vi "SearchPage.vi"() -> ()   [LabVIEW 2016]
uses:
  <resource>/dialog/NewProjectWizard/MetaDataObj/MetaDataObj.lvclass
  <resource>/dialog/NewProjectWizard/Operation to Log.ctl
  <resource>/dialog/NewProjectWizard/MetaDataObj/Accessors/Read Documentation Path.vi
  <vilib>/Platform/browser.llb/Open URL in Default Browser (path).vi
  <resource>/dialog/NewProjectWizard/MetaDataObj/Accessors/Read Custom VI Mode.vi
  <resource>/dialog/NewProjectWizard/Loading Project Info/NI_NPW_Loading Project Info.lvlib
  <resource>/dialog/NewProjectWizard/Filters/NI_NPW_Filters.lvlib
panel:
  in  "Next":string="下一步" caption="下一步"
  in  "Finish":string="完成" caption="完成"
  in  "Filters":string(tree)="All" caption="过滤"
  in  "Main Next":refnum<vi> caption="主界面下一步"
  in  "Additional Search":string caption="附加搜索"
  in  "Project List":picture caption="项目列表"
  out "Go To Next Page":bool caption="转至下一页"
  in  "Tab Backward To":refnum<vi> caption="按Tab后退至"
  in  "Tab Forward To":refnum<vi> caption="按Tab前进至"
  in  "Default Searchbox Text":string="关键词" caption="默认搜索框文本"
  out "Current Starter Application":refnum<class "MetaDataObj.lvclass"> caption="当前启动应用程序"
  in  "Scrollbar":i32(c297) caption="滚动条"
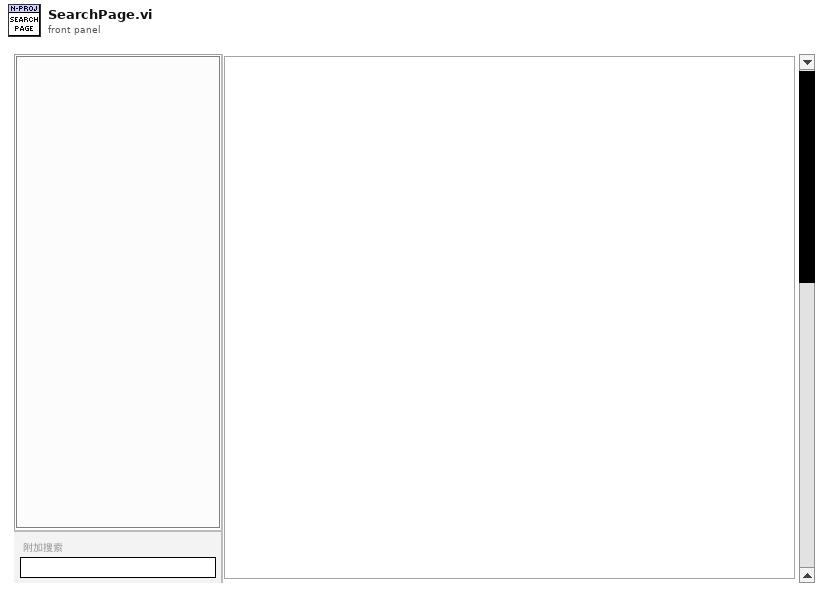
[diagram p1: front panel]
types:
  T1 = typedef "Operation to Log.ctl" = enum16{"Create", "Cancel", "MoreInfoLink"}
  T2 = enum8{"Enabled", "Disabled", "Disabled and Grayed Out"}
  T3 = typedef "imagedata.ctl" = cluster{"image type":i32, "image depth":i32, "image":u8[], "mask":u8[], "colors":u32[], "Rectangle":cluster{"left":i16, "top":i16, "right":i16, "bottom":i16}}
  T4 = typedef "LVBoundsTypeDef.ctl" = cluster{"Width":u32, "Height":u32}
  T5 = typedef "eventvkey.ctl" = enum16{"ASCII", "Enter", "Return", "Shift", "Ctrl", "Alt", "Cmd", "Opt", "Caps", "NumLock", "Clear", "Break", "Up", "Down", "Left", "Right", "Insert", "Delete", "Home", "End", "PageUp", "PageDown", "Escape", "Help", "Pause", "ScrollLock", "F1", "F2", "F3", "F4", "F5", "F6", "F7", "F8", "F9", "F10", "F11", "F12", "F13", "F14", "F15", "F16", "F17", "F18", "F19", "F20", "F21", "F22", "F23", "F24", "Play", "VolumeUp", "VolumeDown", "Mute", "Two Byte Char"}
  T6 = typedef "CustomVIModes.ctl" = enum16{"None", "AfterPage1", "AfterPage2WithUI", "AfterPage2NoUI"}
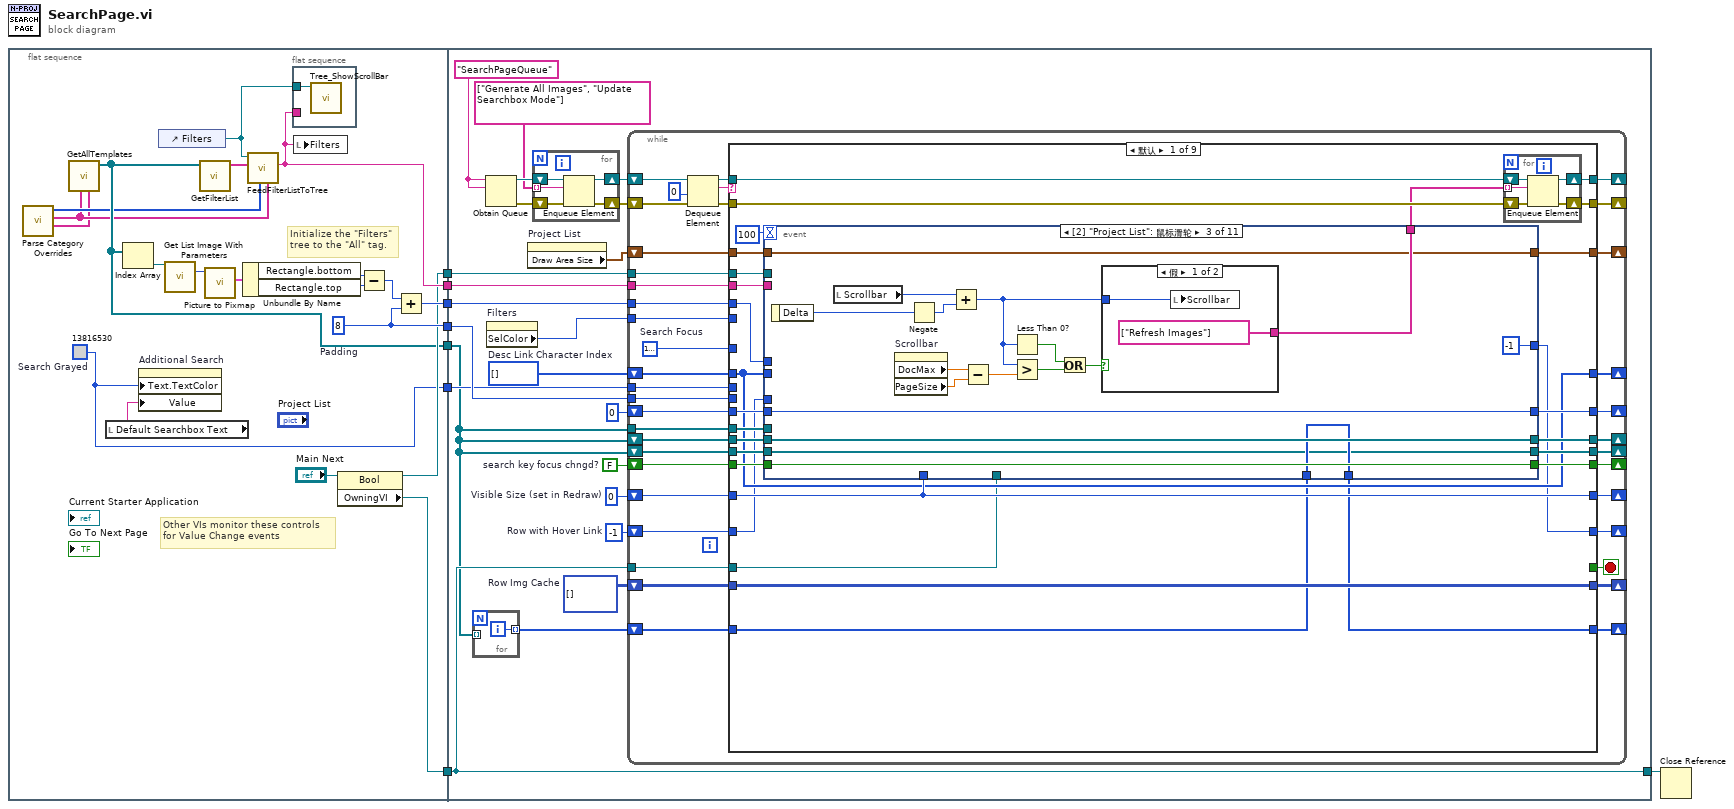
[diagram p0: block diagram]
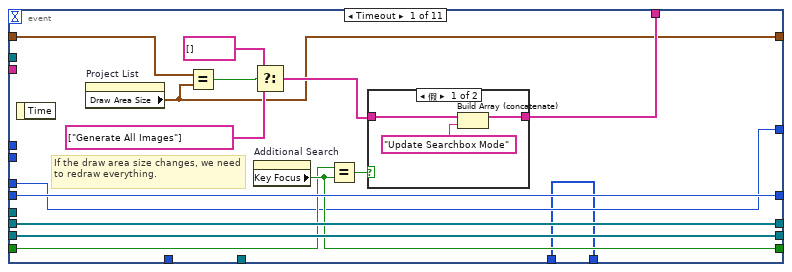
[diagram p2: hidden frame]
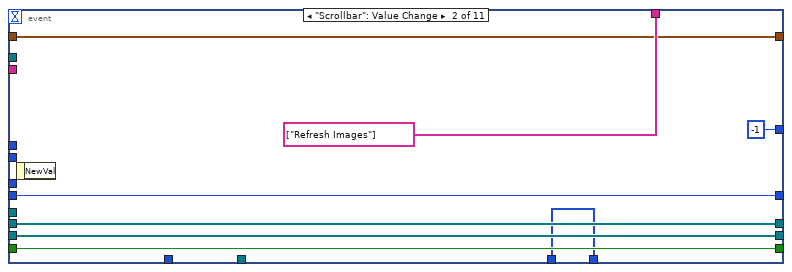
[diagram p4: hidden frame]
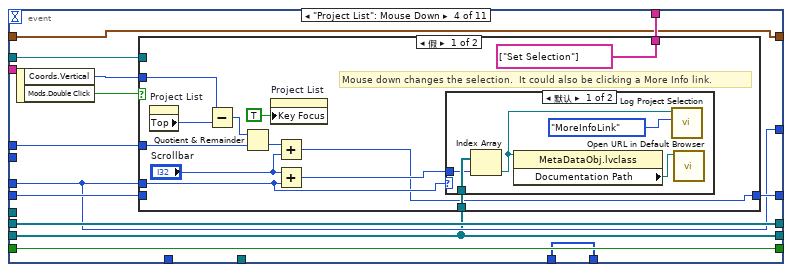
[diagram p6: hidden frame]
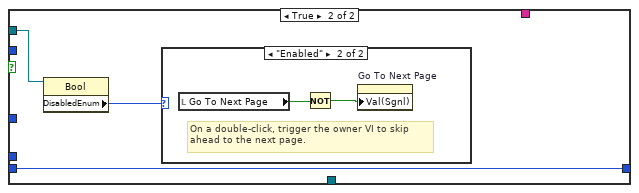
[diagram p8: hidden frame]
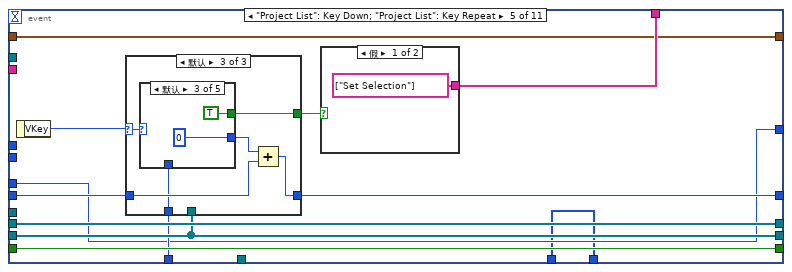
[diagram p10: hidden frame]
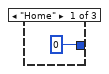
[diagram p12: hidden frame]
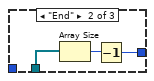
[diagram p13: hidden frame]
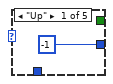
[diagram p14: hidden frame]
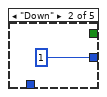
[diagram p15: hidden frame]
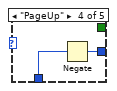
[diagram p16: hidden frame]
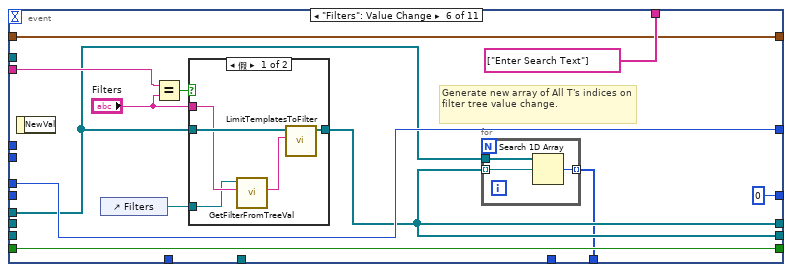
[diagram p18: hidden frame]
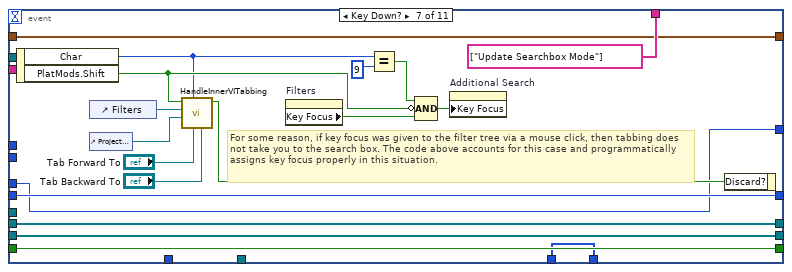
[diagram p20: hidden frame]
diagram:
  n1 = flat-sequence {
    tunnel: [w13] -> w8
    tunnel: [w20] -> w7
    tunnel: [w21] -> w6
    tunnel: [w18] -> w5
    tunnel: [w16] -> w4
    tunnel: [w15] -> w3
    tunnel: [w12] -> w1
    tunnel: w8 -> [w31]
    tunnel: w7 -> [w50]
    tunnel: w6 -> [w49]
    tunnel: w5 -> [w45]
    tunnel: w4 -> [w40]
    tunnel: w3 -> [w39]
    tunnel: [w39] -> w2
    tunnel: w1 -> [w38]
    frame #0 {
      w12 = u32 13816530  # Search Grayed
      w21 = i8 8  # Padding
      # "Other VIs monitor these controls\nfor Value Change events"
      # "Initialize the \"Filters\"\ntree to the \"All\" tag."
      n2 = call <resource>:"Parse Category Overrides.vi"() -> ("Non Localized Names"=w9:string[], "Names"=w10:string[], "Priorities"=w11:i32[])  [unwired: 9 in]
      n3 = call <resource>:"GetAllTemplates.vi"("Category Nonlocalized Names"=w9, "Category Names"=w10) -> ("Templates Out"=w13:refnum<class "MetaDataObj.lvclass">[])  [unwired: 9 in]
      n4 = local read "Default Searchbox Text"() -> (w14:string)
      n5 = Index Array(array=w13) -> (element=w28:refnum<class "MetaDataObj.lvclass">)  [unwired: 1 in]
      n6 = property on="Additional Search" class="Str"("Text.TextColor"=w12, "Value"=w14) -> ()  [unwired: 2 in, 2 out]
      n7 = control-ref of="Filters"() -> (w19:refnum<vi>)
      n8 = call <resource>:"Get List Image With Parameters.vi"("Template in"=w28) -> ("Image"=w27:picture)  [unwired: 10 in, 4 out]
      n9 = call <resource>:"GetFilterList.vi"("Templates"=w13) -> ("Filters"=w23:string[])  [unwired: 10 in]
      n10 = call <vilib>:"Picture to Pixmap.vi"("picture"=w27) -> ("image data"=w26:T3)  [unwired: 9 in, 1 out]
      n11 = Unbundle By Name(w26) -> ("Rectangle.bottom"=w25:i16, "Rectangle.top"=w24:i16)
      n12 = call <resource>:"FeedFilterListToTree.vi"("Category Names"=w10, "Category Priorities"=w11, "Filters"=w23, "Tree Ref In"=w19) -> ("\"All\" Tag"=w20:string)  [unwired: 6 in, 1 out]
      n13 = flat-sequence {
        tunnel: w20 -> [_]
        tunnel: w19 -> [w29]
        frame #0 {
          n14 = call <vilib>:"Tree_ShowScrollBar.vi"("Tree"=w29) -> ()  [unwired: 10 in, 1 out]
        }
      }
      n15 = local write "Filters"(w20) -> ()
      n16 = property class="Bool"(reference="Main Next") -> (reference out=w16:refnum<vi>, "OwningVI"=w15:refnum<vi>)  [unwired: 1 in, 1 out]
      n17 = Subtract(x=w25, y=w24) -> (x-y=w22:i16)
      n18 = Add(x=w22, y=w21) -> (x+y=w18:i16)
    }
    frame #1 {
      w37 = picture[][] []  # Row Img Cache
      w42 = -1  # Row with Hover Link
      w43 = i32[] []  # Desc Link Character Index
      w44 = i8 0  # Visible Size (set in Redraw)
      w46 = FALSE  # search key focus chngd?
      w34 = "SearchPageQueue" ("name (unnamed)")
      n19 = for {
        tunnel: [w52] -> w32 mode=indexing
        tunnel: w31 -> [_] mode=indexing
        i -> [w52]
      }
      n20 = Obtain Queue(name (unnamed)=w34, element data type=w34) -> (queue out=w35:refnum<queue>, error out=w36:errorcluster)  [unwired: 3 in, 1 out]
      n21 = property on="Filters" class="Tree (严格)"() -> ("SelColor"=w41:u32)  [unwired: 2 in, 2 out]
      n22 = property on="Project List" class="Pict"() -> ("Draw Area Size"=w30:T4)  [unwired: 2 in, 2 out]
      n23 = for {
        shift-right: [w57] -> w48
        shift-left: w35 -> [w54]
        shift-right: [w56] -> w47
        shift-left: w36 -> [w55]
        tunnel: string[] ["Generate All Images", "Update Searchbox Mode"] -> [w53] mode=indexing
        n24 = Enqueue Element(queue=w54, element=w53, error in (no error)=w55) -> (queue out=w57:refnum<queue>, error out=w56:errorcluster)  [unwired: 1 in, 1 out]
      }
      n25 = while {
        shift-right: [w90] -> _
        shift-left: w47 -> [w94]
        shift-right: [w78] -> _
        shift-left: w48 -> [w95]
        tunnel: w31 -> [w87]
        shift-right: [w83] -> _
        shift-left: w31 -> [w86]
        shift-right: [w84] -> _
        shift-left: w31 -> [w85]
        shift-right: [w81] -> _
        shift-left: 0 ("Selection") -> [w82]
        tunnel: w50 -> [w80]
        tunnel: w49 -> [w79]
        shift-right: [w75] -> _
        shift-left: w46 -> [w76]
        tunnel: w45 -> [w74]
        shift-right: [w72] -> _
        shift-left: w44 -> [w73]
        shift-right: [w71] -> _
        shift-left: w43 -> [w70]
        shift-right: [w68] -> _
        shift-left: w42 -> [w69]
        tunnel: w41 -> [w67]
        tunnel: w40 -> [w66]
        tunnel: w39 -> [w65]
        tunnel: w38 -> [w64]
        shift-right: [w62] -> _
        shift-left: w37 -> [w63]
        shift-right: [w60] -> _
        shift-left: w32 -> [w61]
        shift-right: [w58] -> _
        shift-left: w30 -> [w59]
        stop <- w88 stop-if-true
        w77 = u32 16777222  # Search Focus
        n26 = Dequeue Element(queue=w95, timeout in ms (-1)=0, error in (no error)=w94) -> (queue out=w93:refnum<queue>, element=w91:string, error out=w92:errorcluster)  [unwired: 1 out]
        n27 = case shown="默认" w91 {
          tunnel: w93 -> [w114 w354 w389 w430 w464 w496 w516 w546 w577]
          tunnel: w92 -> [w113 w351 w400 w429 w462 w497 w515 w545 w576]
          tunnel: [w112 w352 w390 w429 w461 w487 w515 w545 w576] -> w90
          tunnel: [_ _ _ _ _ _ _ _ TRUE] -> w88
          tunnel: w87 -> [w118 _ w385 _ w443 _ _ _ _]
          tunnel: w86 -> [w122 w349 w396 w428 w454 w492 w514 w552 w575]
          tunnel: w85 -> [w120 w348 w395 w427 w455 w491 w513 w551 w574]
          tunnel: [w119 w348 w395 w427 w442 w491 w513 w551 w574] -> w84
          tunnel: [w121 w349 w396 w428 w454 w492 w514 w552 w575] -> w83
          tunnel: w82 -> [w117 w347 w394 w426 _ w490 w512 w550 w573]
          tunnel: [w116 w347 w394 w426 0 ("lower limit") w489 w512 w550 w573] -> w81
          tunnel: w80 -> [w115 _ _ _ _ _ _ _ _]
          tunnel: w79 -> [_ w346 _ _ _ _ _ _ _]
          tunnel: [w110 w353 w388 w430 w463 w488 w516 w546 w577] -> w78
          tunnel: w77 -> [_ _ _ _ w457 _ _ w544 _]
          tunnel: w76 -> [w109 w345 w393 w425 w453 w486 w511 w543 w572]
          tunnel: [w108 w345 w393 w425 w453 w486 w511 w543 w572] -> w75
          tunnel: w74 -> [w107 w344 _ w424 _ _ _ _ _]
          tunnel: w73 -> [w106 _ w383 w423 w452 w485 w510 w542 w571]
          tunnel: [w106 w343 w383 w423 w452 w485 w510 w542 w571] -> w72
          tunnel: [w105 w331 w382 w422 w451 w484 w509 w541 w570] -> w71
          tunnel: w70 -> [w105 w331 _ w422 w451 w484 w509 w541 w570]
          tunnel: w69 -> [w104 w342 w392 w421 w450 w483 w508 w540 w569]
          tunnel: [w103 w342 w392 w421 w450 w483 w508 w540 w569] -> w68
          tunnel: w66 -> [w101 _ _ _ w448 w480 _ _ _]
          tunnel: w67 -> [_ _ w391 _ _ _ _ _ _]
          tunnel: w65 -> [w102 _ _ _ _ _ _ _ _]
          tunnel: w64 -> [_ _ _ _ _ _ _ w539 _]
          tunnel: w63 -> [w100 w333 _ w419 w444 w478 w507 w538 w568]
          tunnel: [w100 w333 w384 w419 w444 w478 w507 w538 w568] -> w62
          tunnel: w61 -> [w99 w332 w386 w418 _ w477 w506 w537 w567]
          tunnel: [w98 w332 w386 w418 w441 w477 w506 w537 w567] -> w60
          tunnel: w59 -> [w97 w325 w381 w417 w440 w476 w505 w536 w566]
          tunnel: [w96 w325 w381 w417 w440 w476 w505 w536 w566] -> w58
          frame Default {
            n28 = event shown="[2] \"Project List\": 鼠标滑轮" {
              selector: _ -> [_ _ _ _ _ _ _ _ _ _ _]
              dyn-events: _ -> [_ _ _ _ _ _ _ _ _ _ _]
              timeout: 100 -> [_ _ _ _ _ _ _ _ _ _ _]
              tunnel: [w137 string[] ["Refresh Images"] w171 w183 w216 string[] ["Enter Search Text"] string[] ["Update Searchbox Mode"] string[] ["Update Searchbox Mode"] w299 w309 string[] ["Update Searchbox Mode"]] -> w111
              tunnel: w122 -> [w143 w155 w173 w186 w220 _ w277 w287 w294 w316 w324]
              tunnel: [w143 w155 w173 w186 w220 w243 w277 w287 w294 w316 w324] -> w121
              tunnel: [w142 w154 w165 w179 w219 w243 w276 w286 w293 w306 w323] -> w119
              tunnel: w120 -> [w142 w154 w165 w179 w219 _ w276 w286 w293 w306 w323]
              tunnel: w118 -> [_ _ _ _ _ w244 _ _ _ _ _]
              tunnel: w117 -> [w141 w153 w172 w184 w217 _ w275 w288 w295 w315 w322]
              tunnel: [w141 w153 w172 w185 w218 0 ("Selection") w275 w288 w295 w315 w322] -> w116
              tunnel: w115 -> [_ _ _ _ _ w249 _ _ _ _ _]
              tunnel: w109 -> [w139 w151 w170 w182 w215 w247 w273 w285 w292 w314 w320]
              tunnel: [w140 w151 w170 w182 w215 w247 w273 w285 w292 w314 w320] -> w108
              tunnel: w107 -> [_ _ _ w181 _ _ _ _ _ w304 _]
              tunnel: w106 -> [_ _ _ _ w214 _ _ _ _ _ _]
              tunnel: w105 -> [_ _ _ _ _ _ _ _ _ w305 _]
              tunnel: w104 -> [w136 _ _ w180 w213 w245 w270 w284 w291 w307 w319]
              tunnel: [w136 -1 ("Row with Hover Link") -1 ("Row with Hover Link") w180 w213 w245 w270 w284 w291 w308 w319] -> w103
              tunnel: w102 -> [_ _ _ _ _ _ _ _ _ w303 _]
              tunnel: w101 -> [_ _ _ w178 _ _ _ _ _ _ _]
              tunnel: w99 -> [w135 w149 w168 w177 w212 _ w269 w283 w290 w302 w318]
              tunnel: [w135 w149 w168 w177 w212 w242 w269 w283 w290 w302 w318] -> w98
              tunnel: w97 -> [w134 w148 w167 w176 w211 w241 w268 w282 w289 w301 w317]
              tunnel: [w129 w148 w167 w176 w211 w241 w268 w282 w289 w301 w317] -> w96
              event Timeout {
                # "If the draw area size changes, we need to redraw everything."
                n29 = event-data() -> ()  [unwired: 1 in, 1 out]
                n30 = property on="Project List" class="Pict"() -> ("Draw Area Size"=w129:T4)  [unwired: 2 in, 2 out]
                n31 = Equal?(x=w134, y=w129) -> (x = y?=w133:bool)
                n32 = property on="Additional Search" class="Str"() -> ("Key Focus"=w140:bool)  [unwired: 2 in, 2 out]
                n33 = Select(t=string[] [], s=w133, f=string[] ["Generate All Images"]) -> (s? t:f=w131:string[])
                n34 = Equal?(x=w139, y=w140) -> (x = y?=w138:bool)
                n35 = case shown="假" w138 {
                  tunnel: w131 -> [w146 w147]
                  tunnel: [w145 w147] -> w137
                  frame False {
                    n36 = Build Array (concatenate)(w146, "Update Searchbox Mode") -> (w145:string[])
                  }
                  frame True {
                  }
                }
              }
              event "Scrollbar": Value Change {
                n37 = event-data() -> ()  [unwired: 1 in, 1 out]
              }
              event "Project List": Mouse Wheel {
                n38 = event-data() -> ("Delta"=w166:i32)  [unwired: 1 in]
                n39 = local read "Scrollbar"() -> (w163:i32)
                n40 = property on="Scrollbar" class="Scroll (严格)"() -> ("DocMax"=w158:dbl, "PageSize"=w157:dbl)  [unwired: 2 in, 2 out]
                n41 = Negate(x=w166) -> (-x=w161:i32)
                n42 = Add(x=w163, y=w161) -> (x+y=w160:i32)
                n43 = Subtract(x=w158, y=w157) -> (x-y=w156:dbl)
                n44 = Less Than 0?(x=w160) -> (x < 0?=w162:bool)
                n45 = Greater?(x=w160, y=w156) -> (0:w164:bool)
                n46 = Or(x=w162, y=w164) -> (x .or. y?=w159:bool)
                n47 = case shown="假" w159 {
                  tunnel: [string[] ["Refresh Images"] _] -> w171
                  tunnel: w160 -> [w174 _]
                  frame False {
                    n48 = local write "Scrollbar"(w174) -> ()
                  }
                  frame True {
                  }
                }
              }
              event "Project List": Mouse Down {
                n49 = event-data() -> ("Coords.Vertical"=w188:i32, "Mods.Double Click"=w187:bool)  [unwired: 1 in]
                n50 = case shown="假" w187 {
                  tunnel: w188 -> [w200 _]
                  tunnel: [w189 w208] -> w185
                  tunnel: w184 -> [_ w208]
                  tunnel: [string[] ["Set Selection"] _] -> w183
                  tunnel: w181 -> [w194 _]
                  tunnel: w180 -> [w190 _]
                  tunnel: w179 -> [w193 _]
                  tunnel: w178 -> [_ w207]
                  frame False {
                    # "Mouse down changes the selection.  It could also be clicking a More Info link."
                    n51 = property on="Project List" class="Pict"() -> ("Top"=w199:i32)  [unwired: 2 in, 2 out]
                    n52 = Subtract(x=w200, y=w199) -> (x-y=w198:i32)
                    n53 = Quotient & Remainder(x=w198, y=w194) -> (floor(x/y)=w197:i32)  [unwired: 1 out]
                    n54 = property on="Project List" class="Pict"("Key Focus"=TRUE) -> ()  [unwired: 2 in, 2 out]
                    n55 = Add(x=w197, y="Scrollbar") -> (x+y=w189:i32)
                    n56 = Add(x="Scrollbar", y=w190) -> (x+y=w191:i32)
                    n57 = case shown="默认" w190 {
                      tunnel: w193 -> [w205 _]
                      tunnel: w191 -> [w204 _]
                      frame Default {
                        n58 = Index Array(array=w205, index=w204) -> (element=w202:refnum<class "MetaDataObj.lvclass">)
                        n59 = property class="MetaDataObj.lvclass"(reference=w202) -> ("Documentation Path"=w203:path)  [unwired: 1 in, 2 out]
                        n60 = call <resource>:"Log Project Selection.vi"("Operation to Log"=Operation_to_Log."MoreInfoLink", "MetaDataObj in"=w202) -> ()  [unwired: 10 in]
                        n61 = call-poly <vilib>:"Open URL in Default Browser.vi"("path"=w203) -> ()  [unwired: 5 in, 2 out]
                      }
                      frame -1 {
                      }
                    }
                  }
                  frame True {
                    n62 = property class="Bool"(reference=w207) -> ("DisabledEnum"=w206:T2)  [unwired: 1 in, 2 out]
                    n63 = case shown="\"Enabled\"" w206 {
                      frame Default {
                        # "If Next is disabled, don't allow a double-click\nto advance to the next page"
                      }
                      frame "Enabled" {
                        # "On a double-click, trigger the owner VI to skip\nahead to the next page."
                        n64 = local read "Go To Next Page"() -> (w209:bool)
                        n65 = Not(x=w209) -> (.not. x?=w210:bool)
                        n66 = property on="Go To Next Page" class="Bool (严格)"("Val(Sgnl)"=w210) -> ()  [unwired: 2 in, 2 out]
                      }
                    }
                  }
                }
              }
              event "Project List": Key Down; "Project List": Key Repeat {
                n67 = event-data() -> ("VKey"=w222:T5)  [unwired: 1 in]
                n68 = case shown="默认" w222 {
                  selector: w222 -> [_ _ w232]
                  tunnel: [0 w226 w231] -> w218
                  tunnel: [_ _ w230] -> w221
                  tunnel: w219 -> [_ w225 _]
                  tunnel: w217 -> [_ _ w229]
                  tunnel: w214 -> [_ _ w228]
                  frame "Home" {
                  }
                  frame "End" {
                    n69 = Array Size(array=w225) -> (size(s)=w227:i32)
                    n70 = Decrement(x=w227) -> (x-1=w226:i32)
                  }
                  frame Default {
                    n71 = case shown="默认" w232 {
                      tunnel: [-1 1 0 w239 w240] -> w233
                      tunnel: [_ _ TRUE _ _] -> w230
                      tunnel: w228 -> [_ _ _ w238 w240]
                      frame "Up" {
                      }
                      frame "Down" {
                      }
                      frame Default {
                      }
                      frame "PageUp" {
                        n72 = Negate(x=w238) -> (-x=w239:i8)
                      }
                      frame "PageDown" {
                      }
                    }
                    n73 = Add(x=w233, y=w229) -> (x+y=w231:i32)
                  }
                }
                n74 = case shown="假" w221 {
                  tunnel: [string[] ["Set Selection"] _] -> w216
                  frame False {
                  }
                  frame True {
                  }
                }
              }
              event "Filters": Value Change {
                # "Generate new array of All T's indices on filter tree value change."
                n75 = event-data() -> ()  [unwired: 1 in, 1 out]
                n76 = control-ref of="Filters"() -> (w251:refnum<vi>)
                n77 = Equal?(x=w249, y="Filters") -> (x = y?=w252:bool)
                n78 = case shown="假" w252 {
                  tunnel: w244 -> [w260 w261]
                  tunnel: [w259 w261] -> w243
                  tunnel: "Filters" -> [w258 _]
                  tunnel: w251 -> [w257 _]
                  frame False {
                    n79 = call <resource>:"GetFilterFromTreeVal.vi"("Value"=w258, "Tree Ref In"=w257) -> ("Filter"=w256:string)  [unwired: 8 in, 1 out]
                    n80 = call <resource>:"LimitTemplatesToFilter.vi"("Filter"=w256, "Templates In"=w260) -> ("Templates Out"=w259:refnum<class "MetaDataObj.lvclass">[])  [unwired: 9 in]
                  }
                  frame True {
                  }
                }
                n81 = for {
                  tunnel: w244 -> [w255]
                  tunnel: w243 -> [w254] mode=indexing
                  tunnel: [w253] -> w242 mode=indexing
                  n82 = Search 1D Array(1D array=w255, element=w254) -> (index of element=w253:i32)  [unwired: 1 in]
                }
              }
              event Key Down? {
                # "For some reason, if key focus was given to the filter tree via a mouse click, then tabbing does not take you to the search box. The code above accounts for this case and programmatically assigns key focus properly in this situation."
                n83 = event-data() -> ("Char"=w264:i16, "PlatMods.Shift"=w266:bool)  [unwired: 1 in]
                n84 = control-ref of="Filters"() -> (w279:refnum<vi>)
                n85 = control-ref of="Project List"() -> (w278:refnum<vi>)
                n86 = call <resource>:"HandleInnerVITabbing.vi"("Tab Backward To"="Tab Backward To", "Tab Forward To"="Tab Forward To", "Char"=w264, "Last Control"=w278, "First Control"=w279, "Shift"=w266) -> ("Discard"=w280:bool)  [unwired: 5 in]
                n87 = property on="Filters" class="Tree (严格)"() -> ("Key Focus"=w267:bool)  [unwired: 2 in, 2 out]
                n88 = Equal?(x=w264, y=i16 9) -> (x = y?=w262:bool)
                n89 = Compound Arithmetic op=AND(w262, invert w266, w267) -> (w265:bool)
                n90 = property on="Additional Search" class="Str"("Key Focus"=w265) -> ()  [unwired: 2 in, 2 out]
                n91 = event-data("Discard?"=w280) -> ()  [unwired: 1 in, 1 out]
              }
              event Mouse Down {
                n92 = event-data() -> ()  [unwired: 1 in, 3 out]
              }
              event "Additional Search": Value Change {
                n93 = event-data() -> ("NewVal"=w297:string, "OldVal"=w298:string)  [unwired: 1 in]
                n94 = Equal?(x=w297, y=w298) -> (x = y?=w296:bool)
                n95 = case shown="假" w296 {
                  tunnel: [string[] ["Enter Search Text", "Refresh Images"] _] -> w299
                  frame False {
                  }
                  frame True {
                  }
                }
              }
              event "Project List": Mouse Move {
                n96 = event-data() -> ("Coords.Vertical"=w311:i32, "Coords.Horizontal"=w310:i32)  [unwired: 1 in]
                n97 = control-ref of="Scrollbar"() -> (w312:refnum<vi>)
                n98 = control-ref of="Project List"() -> (w313:refnum<vi>)
                n99 = call <resource>:"Handle SearchPage Mouse Move.vi"("Vertical Coordinate"=w311, "Horizontal Coordinate"=w310, "List Item Height"=w304, "Row with Hover Link in"=w307, "Scrollbar Refnum"=w312, "Desc Link Character Index Array"=w305, "Draw Area Size"=w301, "Project List Refnum"=w313, "Searched Templates"=w306, "Main VI Refnum"=w303, "Index into All T's"=w302) -> ("Messages"=w309:string[], "Row with Hover Link out"=w308:i32)  [unwired: 7 in]
              }
              event event #0x40; VI Activation {
                n100 = event-data() -> ()  [unwired: 1 in, 1 out]
              }
            }
            n101 = for {
              shift-right: [w127] -> w110
              shift-left: w114 -> [w128]
              shift-right: [w125] -> w112
              shift-left: w113 -> [w126]
              tunnel: w111 -> [w124] mode=indexing
              n102 = Enqueue Element(queue=w128, element=w124, error in (no error)=w126) -> (queue out=w127:refnum<queue>, error out=w125:errorcluster)  [unwired: 1 in, 1 out]
            }
          }
          frame "Refresh Images" {
            # "Refresh Images - Pull appropriate images out of cache. This happens on search/filter change, list scroll, value change, or link hover/unhover."
            # "If the last item index equals the array size, we drew a garbage image at the end. Remove it."
            # "0 - selected\n1- not selected\n2 - selected (hover)\n3 - not selected (hover)"
            # "If number of items is less than capacity of list,\ndraw the whole list"
            n103 = Unbundle By Name(w325) -> ("Height"=w356:u32)
            n104 = Array Size(array=w348) -> (size(s)=w329:i32)
            n105 = Divide(x=w356, y=w344) -> (x/y=w335:dbl)
            n106 = Round Toward -Infinity(1:w335) -> (0:w339:dbl)
            n107 = Less?(x=w329, y=w335) -> (x < y?=w334:bool)
            n108 = Round Toward +Infinity(x=w335) -> (ceil(x): smallest int >= x=w340:dbl)
            n109 = property on="Scrollbar" class="Scroll (严格)"("DocMax"=w329, "PageSize"=w339) -> ("Value"=w338:i32)  [unwired: 2 in, 2 out]
            n110 = Max & Min(x=w340, y=w329) -> (min(x,y)=w355:dbl)  [unwired: 1 out]
            n111 = Select(t=0, s=w334, f=w338) -> (s? t:f=w337:i32)
            n112 = for {
              N: w355 -> [_]
              tunnel: w337 -> [w372]
              tunnel: w347 -> [w371]
              tunnel: [w364] -> w327 mode=indexing
              tunnel: w342 -> [w369]
              tunnel: w333 -> [w367]
              tunnel: w332 -> [w368]
              tunnel: [w360] -> w330
              i -> [w370]
              n113 = Add(x=w370, y=w372) -> (x+y=w360:i32)
              n114 = Equal?(x=w360, y=w371) -> (x = y?=w362:bool)
              n115 = Index Array(array=w368, index=w360) -> (element=w366:i32)
              n116 = Equal?(x=w370, y=w369) -> (x = y?=w363:bool)
              n117 = Index Array(array=w367, index (row)=w366) -> (element=w365:picture[])  [unwired: 1 in]
              n118 = case shown="真" w363 {
                tunnel: w362 -> [w374 w378]
                tunnel: [w373 w377] -> w361
                frame False {
                  n119 = case shown="真" w374 {
                    tunnel: [1 0] -> w373
                    frame False {
                    }
                    frame True {
                    }
                  }
                }
                frame True {
                  n120 = case shown="真" w378 {
                    tunnel: [3 2] -> w377
                    frame False {
                    }
                    frame True {
                    }
                  }
                }
              }
              n121 = Index Array(array=w365, index=w361) -> (element=w364:picture)
            }
            n122 = Equal?(x=w329, y=w330) -> (x = y?=w328:bool)
            n123 = case shown="真" w328 {
              tunnel: w327 -> [w357 w359]
              tunnel: [w357 w358] -> w326
              frame False {
              }
              frame True {
                n124 = Delete From Array(array=w359) -> (array with subset deleted=w358:picture[])  [unwired: 2 in, 1 out]
              }
            }
            n125 = call <resource>:"Stack Images.vi"("Padding"=w346, "Array"=w326) -> ("empty picture"=w341:picture)  [unwired: 9 in]
            n126 = local write "Project List"(w341) -> ()
            n127 = To Byte Integer(number=w340) -> (8bit integer=w343:i8)
            n128 = Enqueue Element(queue=w354, element="Check Listbox Scrollbar", error in (no error)=w351) -> (queue out=w353:refnum<queue>, error out=w352:errorcluster)  [unwired: 1 in, 1 out]
          }
          frame "Generate All Images" {
            # "Generate All Images - Create entire Row Image Cache. This happens only on init or window resize."
            # "0 - selected\n1- not selected\n2 - selected (hover)\n3 - not selected (hover)"
            n129 = Unbundle By Name(w381) -> ("Width"=w399:u32)
            n130 = Subtract(x=w399, y=u32 5) -> (x-y=w397:u32)
            n131 = for {
              tunnel: [w409] -> w384 mode=indexing
              tunnel: w385 -> [w407] mode=indexing
              tunnel: w397 -> [w408]
              tunnel: w391 -> [w406]
              tunnel: [w401] -> w382 mode=indexing
              w402 = bool[] [FALSE, FALSE, TRUE, TRUE]  # Link Hover?
              w403 = bool[] [TRUE, FALSE, TRUE, FALSE]  # Selected?
              w405 = u32 16777215
              n132 = Build Array(w406, w405, w406, w405) -> (w404:u32[])
              n133 = for {
                tunnel: [w416] -> w409 mode=indexing
                tunnel: w408 -> [w415]
                tunnel: w407 -> [w414]
                tunnel: w404 -> [w413] mode=indexing
                tunnel: w403 -> [w412] mode=indexing
                tunnel: w402 -> [w411] mode=indexing
                tunnel: [w410] -> w401
                n134 = call <resource>:"Get List Image With Parameters.vi"("Template in"=w414, "Img Width"=w415, "Background Color"=w413, "Highlight?"=w412, "Underline Link?"=w411) -> ("Image"=w416:picture, "End of Desc Character"=w410:i32)  [unwired: 6 in, 3 out]
              }
            }
            n135 = Enqueue Element(queue=w389, element="Set Selection", error in (no error)=w400) -> (queue out=w388:refnum<queue>, error out=w390:errorcluster)  [unwired: 1 in, 1 out]
          }
          frame "Check Listbox Scrollbar" {
            n136 = Array Size(array=w427) -> (size(s)=w433:i32)
            n137 = Unbundle By Name(w417) -> ("Height"=w431:u32)
            n138 = Multiply(x=w424, y=w433) -> (x*y=w432:i32)
            n139 = Greater?(x=w432, y=w431) -> (0:w420:bool)
            n140 = case shown="假" w420 {
              frame True {
                n141 = property on="Scrollbar" class="Scroll (严格)"("DisabledEnum"=T2."Enabled" ("Disabled")) -> ()  [unwired: 2 in, 2 out]
              }
              frame False {
                n142 = property on="Scrollbar" class="Scroll (严格)"("DisabledEnum"=T2."Disabled and Grayed Out" ("Disabled")) -> (error out=w435:errorcluster, "Value"=w436:i32)  [unwired: 2 in, 1 out]
                n143 = case shown="默认" w436 {
                  tunnel: w435 -> [w439 _]
                  frame Default {
                    n144 = property on="Scrollbar" class="Scroll (严格)"(error in=w439, "Val(Sgnl)"=0 ("Value (Signaling)")) -> ()  [unwired: 1 in, 2 out]
                  }
                  frame 0 {
                  }
                }
              }
            }
          }
          frame "Enter Search Text" {
            # "Generate new array of All T's indices on search value change."
            # "Disable 'Next' if the list is empty"
            n145 = property on="Additional Search" class="Str"() -> ("Text.TextColor"=w458:u32)  [unwired: 2 in, 2 out]
            n146 = Equal?(x=w457, y=w458) -> (x = y?=w456:bool)
            n147 = case shown="真" w456 {
              tunnel: [w468 w470] -> w442
              tunnel: w454 -> [_ w471]
              tunnel: w455 -> [w468 _]
              frame False {
              }
              frame True {
                n148 = case shown="默认" "Additional Search" {
                  selector: "Additional Search" -> [w473 _]
                  tunnel: w471 -> [w474 w475]
                  tunnel: [w472 w475] -> w470
                  frame Default {
                    n149 = call <resource>:"SearchTemplates.vi"("Search Text"=w473, "Filtered Templates"=w474) -> ("Display Templates"=w472:refnum<class "MetaDataObj.lvclass">[])  [unwired: 9 in]
                  }
                  frame "" {
                  }
                }
              }
            }
            n150 = Empty Array?(array=w442) -> (empty?=w449:bool)
            n151 = for {
              tunnel: w443 -> [w467]
              tunnel: w442 -> [w466] mode=indexing
              tunnel: [w465] -> w441 mode=indexing
              n152 = Search 1D Array(1D array=w467, element=w466) -> (index of element=w465:i32)  [unwired: 1 in]
            }
            n153 = Select(t=u8 2, s=w449, f=u8 0) -> (s? t:f=w445:u8)
            n154 = property class="Bool"(reference=w448, "DisabledEnum"=w445) -> ()  [unwired: 1 in, 2 out]
            n155 = Enqueue Element(queue=w464, element="Set Selection", error in (no error)=w462) -> (queue out=w463:refnum<queue>, error out=w461:errorcluster)  [unwired: 1 in, 1 out]
          }
          frame "Set Selection" {
            # "Set Selection runs first, and is used to show the\nappropriate boolean text on the next button"
            n156 = Array Size(array=w491) -> (size(s)=w493:i32)
            n157 = Decrement(x=w493) -> (x-1=w494:i32)
            n158 = Enqueue Element(queue=w496, element="Scroll to Selection", error in (no error)=w497) -> (queue out=w499:refnum<queue>, error out=w498:errorcluster)  [unwired: 1 in, 1 out]
            n159 = In Range and Coerce(upper limit=w494, x=w490, lower limit=0) -> (coerced(x)=w489:i32)  [unwired: 1 out]
            n160 = Index Array(array=w491, index=w489) -> (element=w482:refnum<class "MetaDataObj.lvclass">)
            n161 = property class="MetaDataObj.lvclass"(reference=w482) -> ("Custom VI Mode"=w481:T6)  [unwired: 1 in, 2 out]
            n162 = property on="Current Starter Application" class="LVClassControl (严格)"("Val(Sgnl)"=w482) -> ()  [unwired: 2 in, 2 out]
            n163 = Enqueue Element(queue=w499, element="Refresh Images", error in (no error)=w498) -> (queue out=w488:refnum<queue>, error out=w487:errorcluster)  [unwired: 1 in, 1 out]
            n164 = case shown="\"AfterPage1\"" w481 {
              tunnel: ["Next" "Finish"] -> w479
              frame Default {
              }
              frame "AfterPage1" {
              }
            }
            n165 = property class="Bool"(reference=w480, "BoolText.Text"=w479) -> ()  [unwired: 1 in, 2 out]
          }
          frame "Scroll to Selection" {
            n166 = local read "Scrollbar"() -> (w517:i32)
            n167 = Add(x=w510, y=w517) -> (x+y=w504:i32)
            n168 = In Range and Coerce(upper limit=w504, x=w512, lower limit=w517) -> (In Range?=w518:bool)  [unwired: 1 out]
            n169 = case "Within range?" shown="真" w518 {
              tunnel: w512 -> [w521 w533]
              tunnel: w517 -> [w523 w529]
              tunnel: w510 -> [w520 _]
              tunnel: w504 -> [_ w531]
              frame False {
                n170 = Greater?(x=w521, y=w523) -> (0:w522:bool)
                n171 = case "Scroll down?" shown="真" w522 {
                  tunnel: w521 -> [w524 w527]
                  tunnel: w520 -> [_ w526]
                  tunnel: [w524 w525] -> w519
                  frame False {
                  }
                  frame True {
                    n172 = Subtract(x=w527, y=w526) -> (x-y=w528:i32)
                    n173 = Increment(x=w528) -> (x+1=w525:i32)
                  }
                }
                n174 = local write "Scrollbar"(w519) -> ()
              }
              frame True {
                # "If the selected value+1 is equal to the biggest possible list value, then increment the scrollbar value by one to make sure it is scrolled all the way to the bottom. This ensures the last item is fully visible."
                n175 = Increment(x=w533) -> (x+1=w532:i32)
                n176 = Equal?(x=w531, y=w532) -> (x = y?=w530:bool)
                n177 = case shown="真" w530 {
                  tunnel: w529 -> [_ w535]
                  frame False {
                  }
                  frame True {
                    n178 = Increment(x=w535) -> (x+1=w534:i32)
                    n179 = local write "Scrollbar"(w534) -> ()
                  }
                }
              }
            }
          }
          frame "Update Searchbox Mode" {
            n180 = property on="Additional Search" class="Str"() -> ("Text.Text"=w547:string, "Key Focus"=w549:bool, "Text.TextColor"=w553:u32)  [unwired: 2 in, 2 out]
            n181 = Equal?(x=w553, y=w544) -> (x = y?=w548:bool)
            n182 = case "Has focus text-color?" shown="真" w548 {
              tunnel: w549 -> [w556 w563]
              tunnel: w547 -> [w555 w562]
              tunnel: w544 -> [_ w561]
              tunnel: w539 -> [w554 _]
              frame True {
                n183 = case "Has key focus?" shown="假" w556 {
                  tunnel: w555 -> [w558 _]
                  tunnel: w554 -> [w557 _]
                  frame False {
                    n184 = case shown="\"\"" w558 {
                      tunnel: w557 -> [_ w559]
                      frame Default {
                      }
                      frame "" {
                        n185 = property on="Additional Search" class="Str"("Text.TextColor"=w559, "Value"="Default Searchbox Text") -> ()  [unwired: 2 in, 2 out]
                      }
                    }
                  }
                  frame True {
                  }
                }
              }
              frame False {
                n186 = case "Has key focus?" shown="真" w563 {
                  tunnel: w562 -> [_ _]
                  tunnel: w561 -> [_ w565]
                  frame False {
                  }
                  frame True {
                    n187 = property on="Additional Search" class="Str"("Text.TextColor"=w565, "Value"="") -> ()  [unwired: 2 in, 2 out]
                  }
                }
              }
            }
          }
          frame "Quit" {
          }
        }
      }
    }
  }
  n188 = Close Reference(reference=w2) -> ()  [unwired: 1 in, 1 out]
